vi "getEvaluation.vi"(8 "error in (no error)":errorcluster, 11 "GraphNode in":refnum<class "GraphNode.lvclass">) -> (0 "error out":errorcluster, 2 "Evaluation":cluster{"F":dbl, "G":dbl, "H":dbl}, 3 "GraphNode out":refnum<class "GraphNode.lvclass">)   [LabVIEW 2014, in "Graph.lvlib" / "GraphNode.lvclass"]
uses:
  <userlib>/AdvancedDataStructures/ClassBased/GraphNode/GraphNode.lvclass
  <userlib>/AdvancedDataStructures/ClassBased/GraphNode/GraphNode.lvclass/GraphNode.ctl
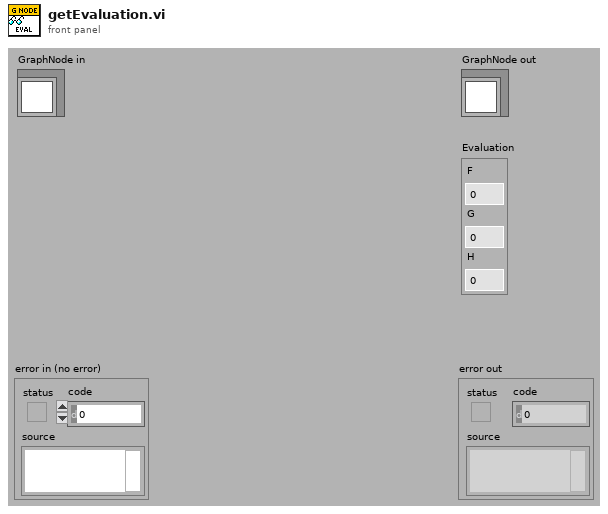
[diagram p1: front panel]
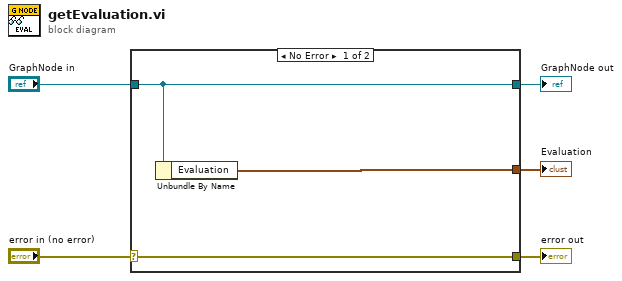
[diagram p0: block diagram]
diagram:
  n1 = case shown="No Error" "error in (no error)" {
    selector: "error in (no error)" -> [w8 w9]
    tunnel: [w8 w9] -> w4
    tunnel: [w7 w10] -> w2
    tunnel: "GraphNode in" -> [w7 w10]
    tunnel: [w6 _] -> w1
    frame No Error {
      n2 = Unbundle By Name(w7) -> ("Evaluation"=w6:cluster{"F":dbl, "G":dbl, "H":dbl})
    }
    frame Error {
    }
  }
  "error out" <- w4
  "GraphNode out" <- w2
  "Evaluation" <- w1
